vi "Set Cell Type (Cell).vi"(7 "Cell Type":T1=1 items=["Numeric"=0, "String"=1, "Formula"=2, "Blank"=3, "Boolean"=4, "Error"=5, "Unknown"=-1], 8 "error in (no error)":errorcluster, 10 "ICell Reference":refnum<k24>) -> (0 "error out":errorcluster, 2 "ICell Reference":refnum<k24>)   [LabVIEW 2013]
uses:
  C:/PhaeronGit/LVNPOI/Resources/NPOI 2.1.1 dotnet2/NPOI.dll
  Resources/NPOI 2.1.1 dotnet2/NPOI.dll
  Typedefs/Cell Types.ctl
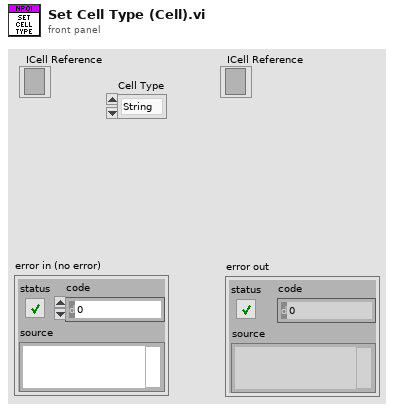
[diagram p1: front panel]
types:
  T1 = typedef "Cell Types.ctl" = i32
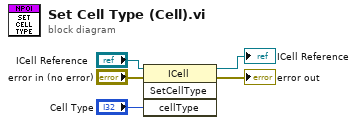
[diagram p0: block diagram]
diagram:
  n1 = invoke class="ICell" method="SetCellType"(reference="ICell Reference", error in="error in (no error)", "cellType"="Cell Type") -> (reference out=→"ICell Reference":refnum<k24>, error out=→"error out":errorcluster)  [unwired: 1 in, 2 out]
